vi "DB_Global_4_kart-Test.vi"() -> ()   [LabVIEW 2014]
panel:
  in  "Manuel Kullan":bool
  in  "phase 5/1":dbl format="%0.5p"
  in  "amplitude 5/1":dbl=1.0 format="%0.5p"
  in  "phase 5/0":dbl format="%0.5p"
  in  "amplitude 5/0":dbl=1.0 format="%0.5p"
  in  "Input.BufSize":u32=200000 format="%.0p"
  in  "Frequency":dbl=1000.0
  in  "phase 3/1":dbl format="%0.5p"
  in  "amplitude 3/1":dbl=1.0 format="%0.5p"
  in  "phase 3/0":dbl format="%0.5p"
  in  "amplitude 3/0":dbl=1.0 format="%0.5p"
  in  "phase 2/1":dbl format="%0.5p"
  in  "amplitude 2/1":dbl=1.0 format="%0.5p"
  in  "phase 2/ 0":dbl format="%0.5p"
  in  "amplitude 2/0":dbl=1.0 format="%0.5p"
  in  "phase 1/1":dbl format="%0.5p"
  in  "amplitude 1/1":dbl=1.0 format="%0.5p"
  in  "phase 1/ 0":dbl format="%0.5p"
  in  "amplitude 1/0":dbl=1.0 format="%0.5p"
  # "Channel Settings"
  # "10R VH"
  # "Besleme"
  # "Ana Denge"
  # "Wagner"
  # "Kelvin"
  # "1R VH"
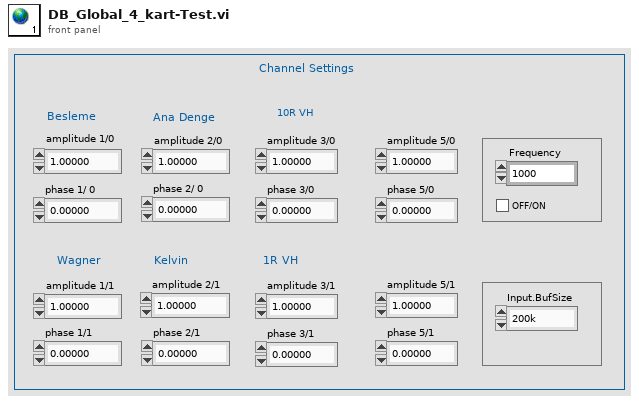
[diagram p1: front panel]
diagram:
